vi "Set DefaultValue.vi"(8 "error in":errorcluster, 10 "Value":refnum<class "Value.lvclass">, 11 "Object Type in":refnum<class "Object Type Base.lvclass">) -> (0 "error out":errorcluster, 3 "Object Type out":refnum<class "Object Type Base.lvclass">)   [LabVIEW 2019, in "Electronic Datasheet.lvlib" / "Object Type Base.lvclass"]
uses:
  Object Type Base.lvclass
  Value/Value.lvclass
  Object Type Base.lvclass/Object Type Base.ctl
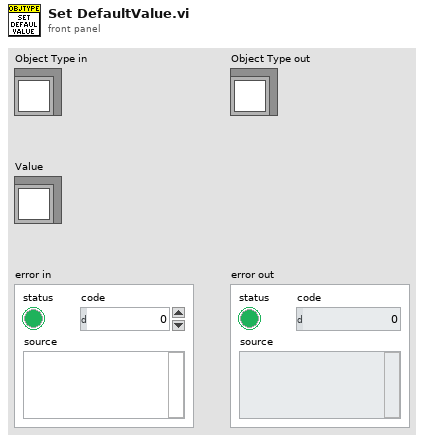
[diagram p1: front panel]
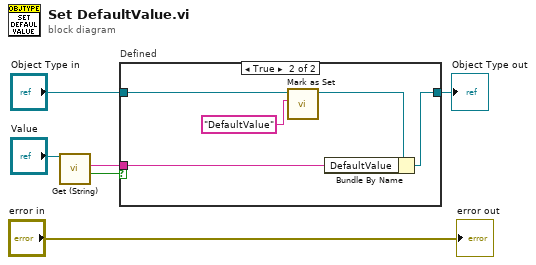
[diagram p0: block diagram]
diagram:
  n1 = call "Get (String).vi"("Value in"="Value") -> ("Defined?"=w3:bool, "Value"=w2:string)  [unwired: 8 in, 1 out]
  n2 = case "Defined" shown="True" w3 {
    tunnel: [w7 w12] -> w6
    tunnel: "Object Type in" -> [w7 w11]
    tunnel: w2 -> [_ w8]
    frame False {
    }
    frame True {
      n3 = call "Mark as Set.vi"("Field name"="DefaultValue" ("element"), "Object Type in"=w11) -> ("Object Type out"=w10:refnum<class "Object Type Base.lvclass">)  [unwired: 9 in]
      n4 = Bundle By Name(cluster=w10, "DefaultValue"=w8) -> (w12:refnum<class "Object Type Base.lvclass">)
    }
  }
  "Object Type out" <- w6
  "error out" <- "error in"
